vi "Generator_c.vi"(0 "Stop":bool caption="Start/Stop") -> (4 "Generated_Data":dbl caption="Generated Data")   [LabVIEW 2023]
doc: "This VI continuously generate Data and push it to the Acquisition VI.\nTransfer of thet data happens under Queue LV2."
uses:
  Type_Def/Operation_Queue.ctl
  <vilib>/numeric/Random Number (Range) DBL.vi
panel:
  out "Error_Out":errorcluster
  in  "Error_In":errorcluster
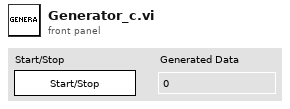
[diagram p1: front panel]
types:
  T1 = typedef "Operation_Queue.ctl" = enum16{"Initialize", "Enqueue", "Dequeue", "Sum"}
  T2 = enum16{"Left Button", "Center Button", "Right Button", "Window Close"}
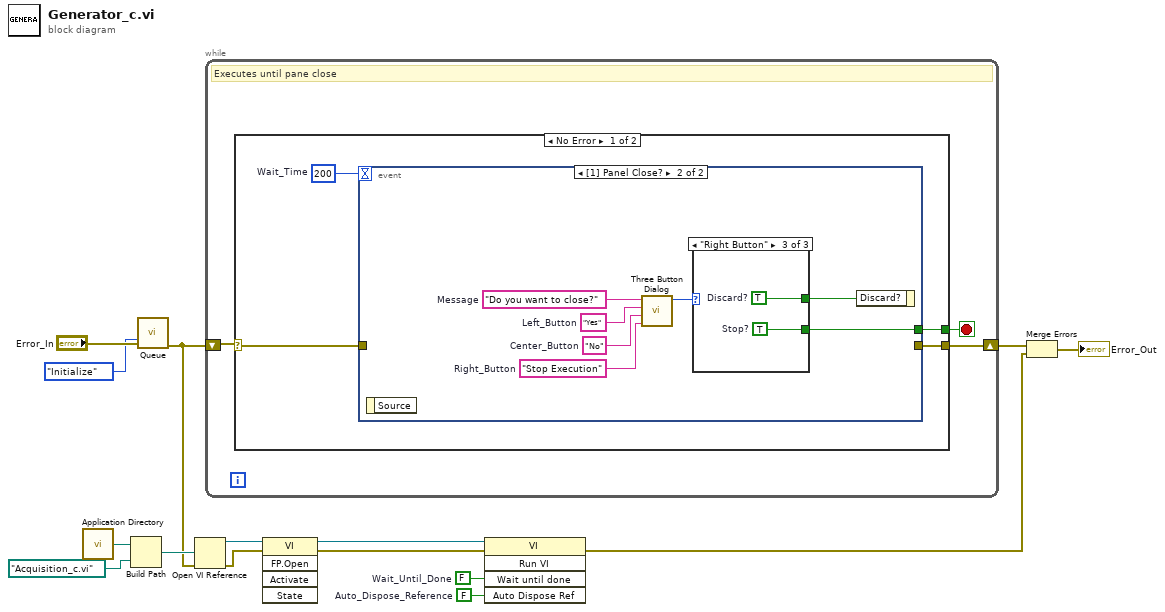
[diagram p0: block diagram]
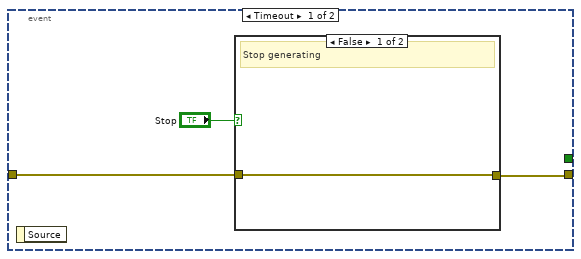
[diagram p2: hidden frame]
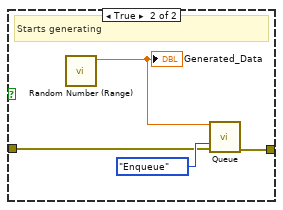
[diagram p3: hidden frame]
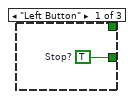
[diagram p4: hidden frame]
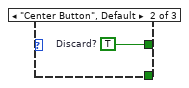
[diagram p5: hidden frame]
diagram:
  w6 = FALSE  # Auto_Dispose_Reference
  w7 = FALSE  # Wait_Until_Done
  n1 = call <vilib>:"Application Directory.vi"() -> ("Application Directory"=w12:path)
  n2 = Build Path(base path=w12, name or relative path=path "Acquisition_c.vi") -> (appended path=w11:path)
  n3 = call "Queue.vi"("Operation"=Operation_Queue."Initialize" ("Operation_Queue"), "Error_In"="Error_In") -> ("Error_Out"=w1:errorcluster)  [unwired: 9 in, 4 out]
  n4 = Open VI Reference(vi path=w11, error in (no error)=w1) -> (vi reference=w9:refnum<vi>, error out=w2:errorcluster)  [unwired: 4 in]
  n5 = while {
    shift-right: [w16] -> w15
    shift-left: w1 -> [w17]
    stop <- w18 stop-if-true
    # "Executes until pane close"
    n6 = case shown="No Error" w17 {
      selector: w17 -> [w20 w42]
      tunnel: [w21 _] -> w18
      tunnel: [w19 w42] -> w16
      frame No Error {
        w22 = 200  # Wait_Time
        n7 = event shown="[1] Panel Close?" {
          selector: _ -> [_ _]
          dyn-events: _ -> [_ _]
          timeout: w22 -> [_ _]
          tunnel: [_ w31] -> w21
          tunnel: w20 -> [w23 _]
          tunnel: [w24 _] -> w19
          event Timeout {
            n8 = event-data() -> ()  [unwired: 1 in, 1 out]
            n9 = case shown="False" "Stop" {
              tunnel: w23 -> [w26 w27]
              tunnel: [w26 w30] -> w24
              frame False {
                # "Stop generating"
              }
              frame True {
                # "Starts generating"
                n10 = call-poly <vilib>:"Random Number (Range).vi"() -> ("number"=w29:dbl)  [unwired: 11 in]
                "Generated_Data" <- w29
                n11 = call "Queue.vi"("Element_In"=w29, "Operation"=Operation_Queue."Enqueue" ("Operation_Queue"), "Error_In"=w27) -> ("Error_Out"=w30:errorcluster)  [unwired: 8 in, 4 out]
              }
            }
          }
          event Panel Close? {
            w34 = "Stop Execution"  # Right_Button
            w35 = "No"  # Center_Button
            w36 = "Yes"  # Left_Button
            w37 = "Do you want to close?"  # Message
            n12 = event-data() -> ()  [unwired: 1 in, 1 out]
            n13 = call <vilib>:"Three Button Dialog.vi"("Right Button Text (\"Cancel\")"=w34, "Center Button Text (\"No\")"=w35, "Left Button Text (\"Yes\")"=w36, "message"=w37) -> ("Which Button?"=w33:T2)  [unwired: 7 in]
            n14 = case shown="\"Right Button\"" w33 {
              tunnel: [_ w39 w40] -> w32
              tunnel: [w38 _ w41] -> w31
              frame "Left Button" {
                w38 = TRUE  # Stop?
              }
              frame "Center Button", Default {
                w39 = TRUE  # Discard?
              }
              frame "Right Button" {
                w40 = TRUE  # Discard?
                w41 = TRUE  # Stop?
              }
            }
            n15 = event-data ("Event Filter Node")("Discard?"=w32) -> ()  [unwired: 1 in, 1 out]
          }
        }
      }
      frame Error {
      }
    }
  }
  n16 = invoke on="Invoke Node" class="VI" method="FP.Open"(reference=w9, error in=w2) -> (reference out=w8:refnum<vi>, error out=w5:errorcluster)  [unwired: 3 in, 3 out]
  n17 = invoke on="Invoke Node" class="VI" method="Run VI"(reference=w8, error in=w5, "Wait until done"=w7, "Auto Dispose Ref"=w6) -> (error out=w3:errorcluster)  [unwired: 1 in, 4 out]
  n18 = Merge Errors(w15, w3) -> (→"Error_Out":errorcluster)
